vi "ModifyGraph Log.vi"(8 "error in (no error)":errorcluster, 10 "Log":T1, 11 "ITX Commands in":refnum<class "ITX Commands.lvclass">) -> (0 "error out":errorcluster, 3 "ITX Commands out":refnum<class "ITX Commands.lvclass">)   [LabVIEW 2019, in "ITX Commands.lvclass"]
uses:
  ITX Commands.lvclass
  typedefs/log--enum.ctl
  typedefs/Log--cluster.ctl
panel:
  out "resulting string":string
  # "n=0: normal axis\nn=1: log base 10\nn=2: log base 2"
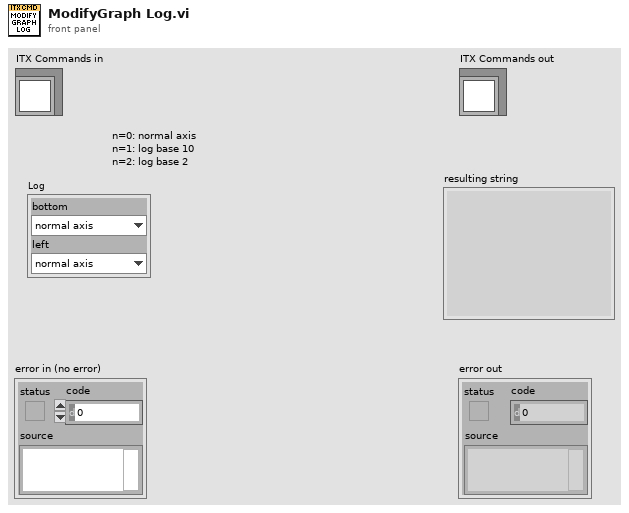
[diagram p1: front panel]
types:
  T1 = typedef "ITX Commands.lvclass/Log--cluster.ctl" = cluster{"bottom":T2, "left":T2}
  T2 = typedef "ITX Commands.lvclass/log--enum.ctl" = enum16{"normal axis", "log base 10", "log base 2"}
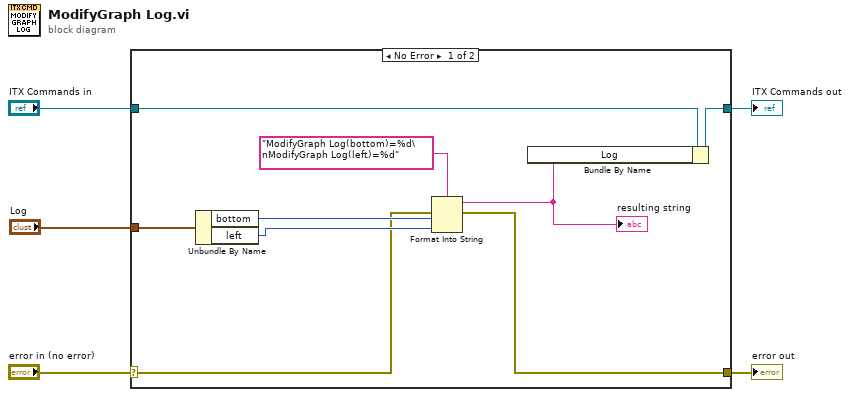
[diagram p0: block diagram]
diagram:
  n1 = case shown="No Error" "error in (no error)" {
    selector: "error in (no error)" -> [w7 w16]
    tunnel: [w6 w16] -> w4
    tunnel: [w9 w15] -> w2
    tunnel: "ITX Commands in" -> [w13 w15]
    tunnel: "Log" -> [w12 _]
    frame No Error {
      n2 = Unbundle By Name(w12) -> ("bottom"=w11:T2, "left"=w10:T2)
      n3 = Format Into String(format string="ModifyGraph Log(bottom)=%d\nModifyGraph Log(left)=%d", error in=w7, w11, w10) -> (resulting string=w8:string, error out=w6:errorcluster)  [unwired: 1 in]
      "resulting string" <- w8
      n4 = Bundle By Name(cluster=w13, "Log"=w8) -> (w9:refnum<class "ITX Commands.lvclass">)
    }
    frame Error {
    }
  }
  "error out" <- w4
  "ITX Commands out" <- w2
